vi "ziSweepUnitConversion.vi"(4 "signal unit":string="V", 6 "Eq Noise BWs (Hz)":dbl[](array[numeric]), 8 "display unit":T2(ring), 9 "log/linear":enum16{"Linear", "dB", "dBm"}(ring)=enum."dB", 10 "spectrum type (Vrms)":T1(ring), 11 "Spectrum in":dbl[](array[numeric])) -> (0 "spectrum unit":string="dBVrms", 3 "Spectrum out":dbl[](array[numeric]))   [LabVIEW 2009, in "Zurich Instruments LabOne.lvlib"]
doc: "Converts either the amplitude or gain (amplitude ratio) spectrum to alternate formats including Log (decibel and dbm) and spectral density."
uses:
  <instrlib>/Zurich Instruments LabOne/Zurich Instruments LabOne.lvlib
panel:
  # "Spectrum Unit Conversion"
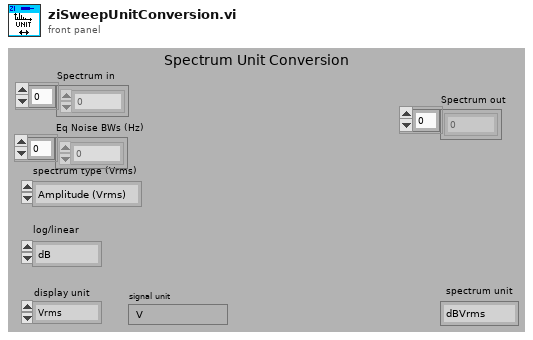
[diagram p1: front panel]
types:
  T1 = enum16{"Amplitude (Vrms)", "Gain (amplitude ratio)"}
  T2 = enum32{"Vrms", "Vpk", "Vrms^2", "Vpk^2", "Vrms/rtHz", "Vpk/rtHz", "Vrms^2/Hz", "Vpk^2/Hz"}
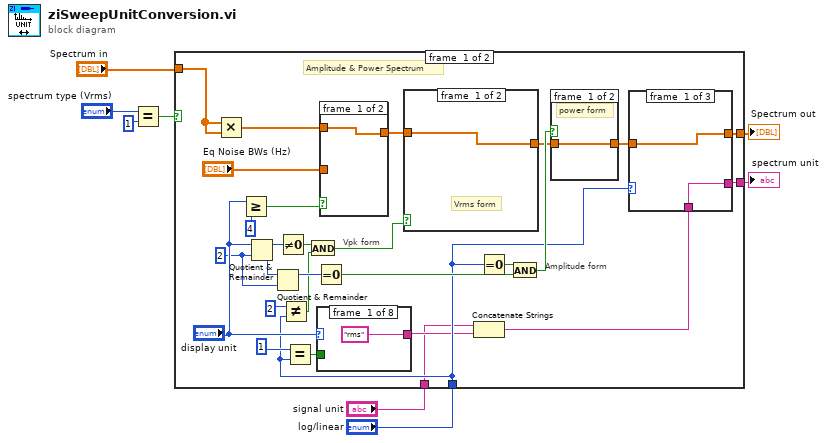
[diagram p0: block diagram]
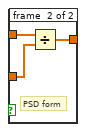
[diagram p2: hidden frame]
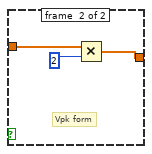
[diagram p3: hidden frame]
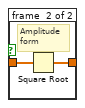
[diagram p4: hidden frame]
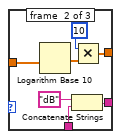
[diagram p5: hidden frame]
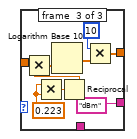
[diagram p6: hidden frame]
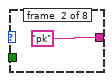
[diagram p7: hidden frame]
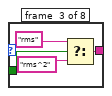
[diagram p8: hidden frame]
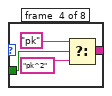
[diagram p9: hidden frame]
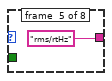
[diagram p10: hidden frame]
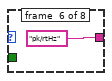
[diagram p11: hidden frame]
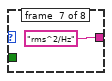
[diagram p12: hidden frame]
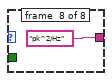
[diagram p13: hidden frame]
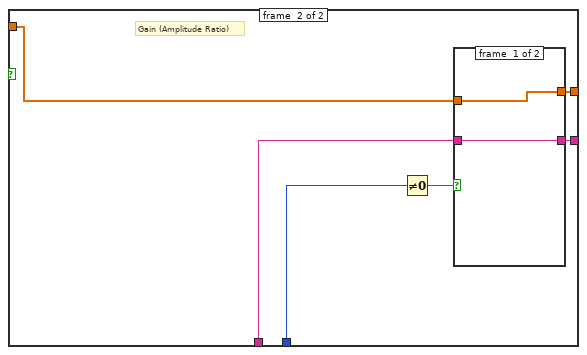
[diagram p14: hidden frame]
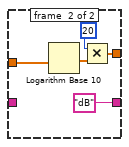
[diagram p15: hidden frame]
diagram:
  n1 = Equal?(x="spectrum type (Vrms)", y=1) -> (x = y?=w7:bool)
  n2 = case shown="False" w7 {
    tunnel: [w24 w85] -> w8
    tunnel: [w23 w84] -> w2
    tunnel: "Spectrum in" -> [w22 w83]
    tunnel: "log/linear" -> [w17 w81]
    tunnel: "signal unit" -> [w9 w80]
    frame #0 {
      w30 = 2
      # "Amplitude & Power Spectrum"
      # "Vpk form"
      # "Amplitude form"
      n3 = Multiply(x=w22, y=w22) -> (x*y=w10:dbl[])
      n4 = Greater Or Equal?(x="display unit", y=4) -> (x >= y?=w26:bool)
      n5 = Quotient & Remainder(x="display unit", y=w30) -> (x-y*floor(x/y)=w27:u32, floor(x/y)=w29:u32)
      n6 = Quotient & Remainder(x=w29, y=w30) -> (x-y*floor(x/y)=w31:u32)  [unwired: 1 out]
      n7 = Not Equal To 0?(x=w27) -> (x != 0?=w15:bool)
      n8 = Not Equal?(x=2, y=w17) -> (x != y?=w16:bool)
      n9 = Equal?(x=1, y=w17) -> (x = y?=w20:bool)
      n10 = And(x=w15, y=w16) -> (x .and. y?=w14:bool)
      n11 = Equal To 0?(x=w31) -> (x = 0?=w19:bool)
      n12 = case shown="..\"Vrms\"" "display unit" {
        tunnel: ["rms" "pk" w71 w75 "rms/rtHz" "pk/rtHz" "rms^2/Hz" "pk^2/Hz"] -> w13
        tunnel: w20 -> [_ _ w70 w74 _ _ _ _]
        frame #0 {
        }
        frame #1 {
        }
        frame #2 {
          n13 = Select(t="rms", s=w70, f="rms^2") -> (s? t:f=w71:string)
        }
        frame #3 {
          n14 = Select(t="pk", s=w74, f="pk^2") -> (s? t:f=w75:string)
        }
        frame #4 {
        }
        frame #5 {
        }
        frame #6 {
        }
        frame #7 {
        }
      }
      n15 = case shown="True" w26 {
        tunnel: [w37 w39] -> w28
        tunnel: "Eq Noise BWs (Hz)" -> [_ w38]
        tunnel: w10 -> [w37 w40]
        frame #0 {
        }
        frame #1 {
          # "PSD form"
          n16 = Divide(x=w40, y=w38) -> (x/y=w39:dbl[])
        }
      }
      n17 = case shown="True" w14 {
        tunnel: [w41 w43] -> w32
        tunnel: w28 -> [w41 w44]
        frame #0 {
          # "Vrms form"
        }
        frame #1 {
          # "Vpk form"
          n18 = Multiply(x=w44, y=2) -> (x*y=w43:dbl[])
        }
      }
      n19 = Concatenate Strings(w9, w13) -> (w12:string)
      n20 = Equal To 0?(x=w17) -> (x = 0?=w36:bool)
      n21 = And(x=w36, y=w19) -> (x .and. y?=w35:bool)
      n22 = case shown="False" w35 {
        tunnel: [w45 w46] -> w33
        tunnel: w32 -> [w45 w47]
        frame #0 {
          # "power form"
        }
        frame #1 {
          # "Amplitude \nform"
          n23 = Square Root(x=w47) -> (sqrt(x)=w46:dbl[])
        }
      }
      n24 = case shown="\"dBm\".." w17 {
        tunnel: w33 -> [w48 w56 w61]
        tunnel: w12 -> [w49 w52 _]
        tunnel: [w49 w51 "dBm"] -> w23
        tunnel: [w48 w50 w63] -> w24
        frame #0 {
        }
        frame #1 {
          n25 = Logarithm Base 10(1:w56) -> (0:w55:dbl[])
          n26 = Concatenate Strings("dB", w52) -> (w51:string)
          n27 = Multiply(x=10, y=w55) -> (x*y=w50:dbl[])
        }
        frame #2 {
          w59 = 0.223
          n28 = Multiply(x=w59, y=w59) -> (x*y=w58:dbl)
          n29 = Reciprocal(x=w58) -> (1/x=w57:dbl)
          n30 = Multiply(x=w61, y=w57) -> (x*y=w62:dbl[])
          n31 = Logarithm Base 10(1:w62) -> (0:w65:dbl[])
          n32 = Multiply(x=10, y=w65) -> (x*y=w63:dbl[])
        }
      }
    }
    frame #1 {
      # "Gain (Amplitude Ratio)"
      n33 = Not Equal To 0?(x=w81) -> (x != 0?=w82:bool)
      n34 = case shown="False" w82 {
        tunnel: [w87 w88] -> w85
        tunnel: w83 -> [w87 w92]
        tunnel: [w86 "dB"] -> w84
        tunnel: w80 -> [w86 _]
        frame #0 {
        }
        frame #1 {
          n35 = Logarithm Base 10(1:w92) -> (0:w91:dbl[])
          n36 = Multiply(x=20, y=w91) -> (x*y=w88:dbl[])
        }
      }
    }
  }
  "spectrum unit" <- w2
  "Spectrum out" <- w8
